vi "UI_Main.vi"(8 "error in (no error)":errorcluster, 11 "Queue Bus":T2) -> (0 "error out":errorcluster)   [LabVIEW 2020]
uses:
  Typedefs/UI_actionButton.ctl
  Typedefs/queueBus.ctl
  Typedefs/communicationData.ctl
  Typedefs/UI_controlRefs.ctl
  Typedefs/enumeratedPlayers.ctl
  Typedefs/gameState.ctl
panel:
  in  "Solve":T1
  out "Puzzle":string
  out "Cash 3":dbl caption="Player 3 cash"
  out "Cash 2":dbl caption="Player 2 cash"
  out "Cash":dbl caption="dddd cash"
  in  "buyVowel":T1
  in  "spin":T1
  out "P3_LED":bool caption="Player 3"
  out "P2_LED":bool caption="Player 2"
  in  "e-stop":bool
  out "P1_LED":bool caption="dddd"
  # "ctrl+x to quit"
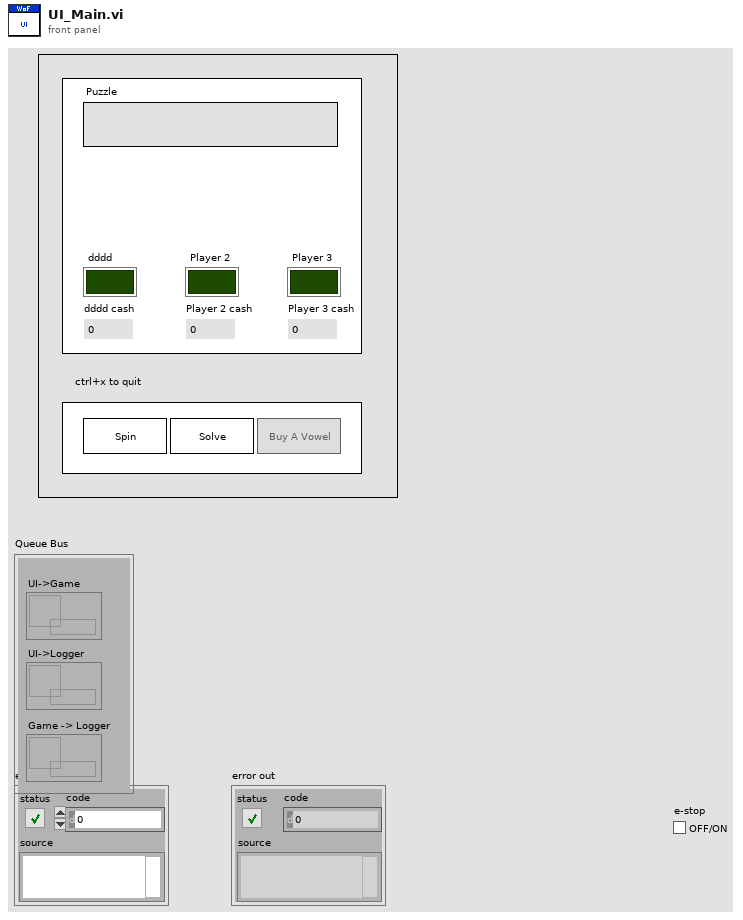
[diagram p1: front panel]
types:
  T1 = typedef "UI_actionButton.ctl" = bool
  T2 = typedef "queueBus.ctl" = cluster{"UI->Game":refnum<queue>, "UI->Logger":refnum<queue>, "Game -> Logger":refnum<queue>}
  T3 = typedef "UI_controlRefs.ctl" = cluster{"spin":refnum<vi>, "buyVowel":refnum<vi>, "Puzzle":refnum<vi>}
  T4 = typedef "communicationData.ctl" = cluster{"command":string, "payload":variant, "response":variant}
  T5 = typedef "enumeratedPlayers.ctl" = enum16{"one", "two", "three"}
  T6 = typedef "gameState.ctl" = cluster{"active player":T5, "Winnings":dbl[], "Vowel Enabled?":bool, "Puzzle State":string, "Puzzle Solved?":bool}
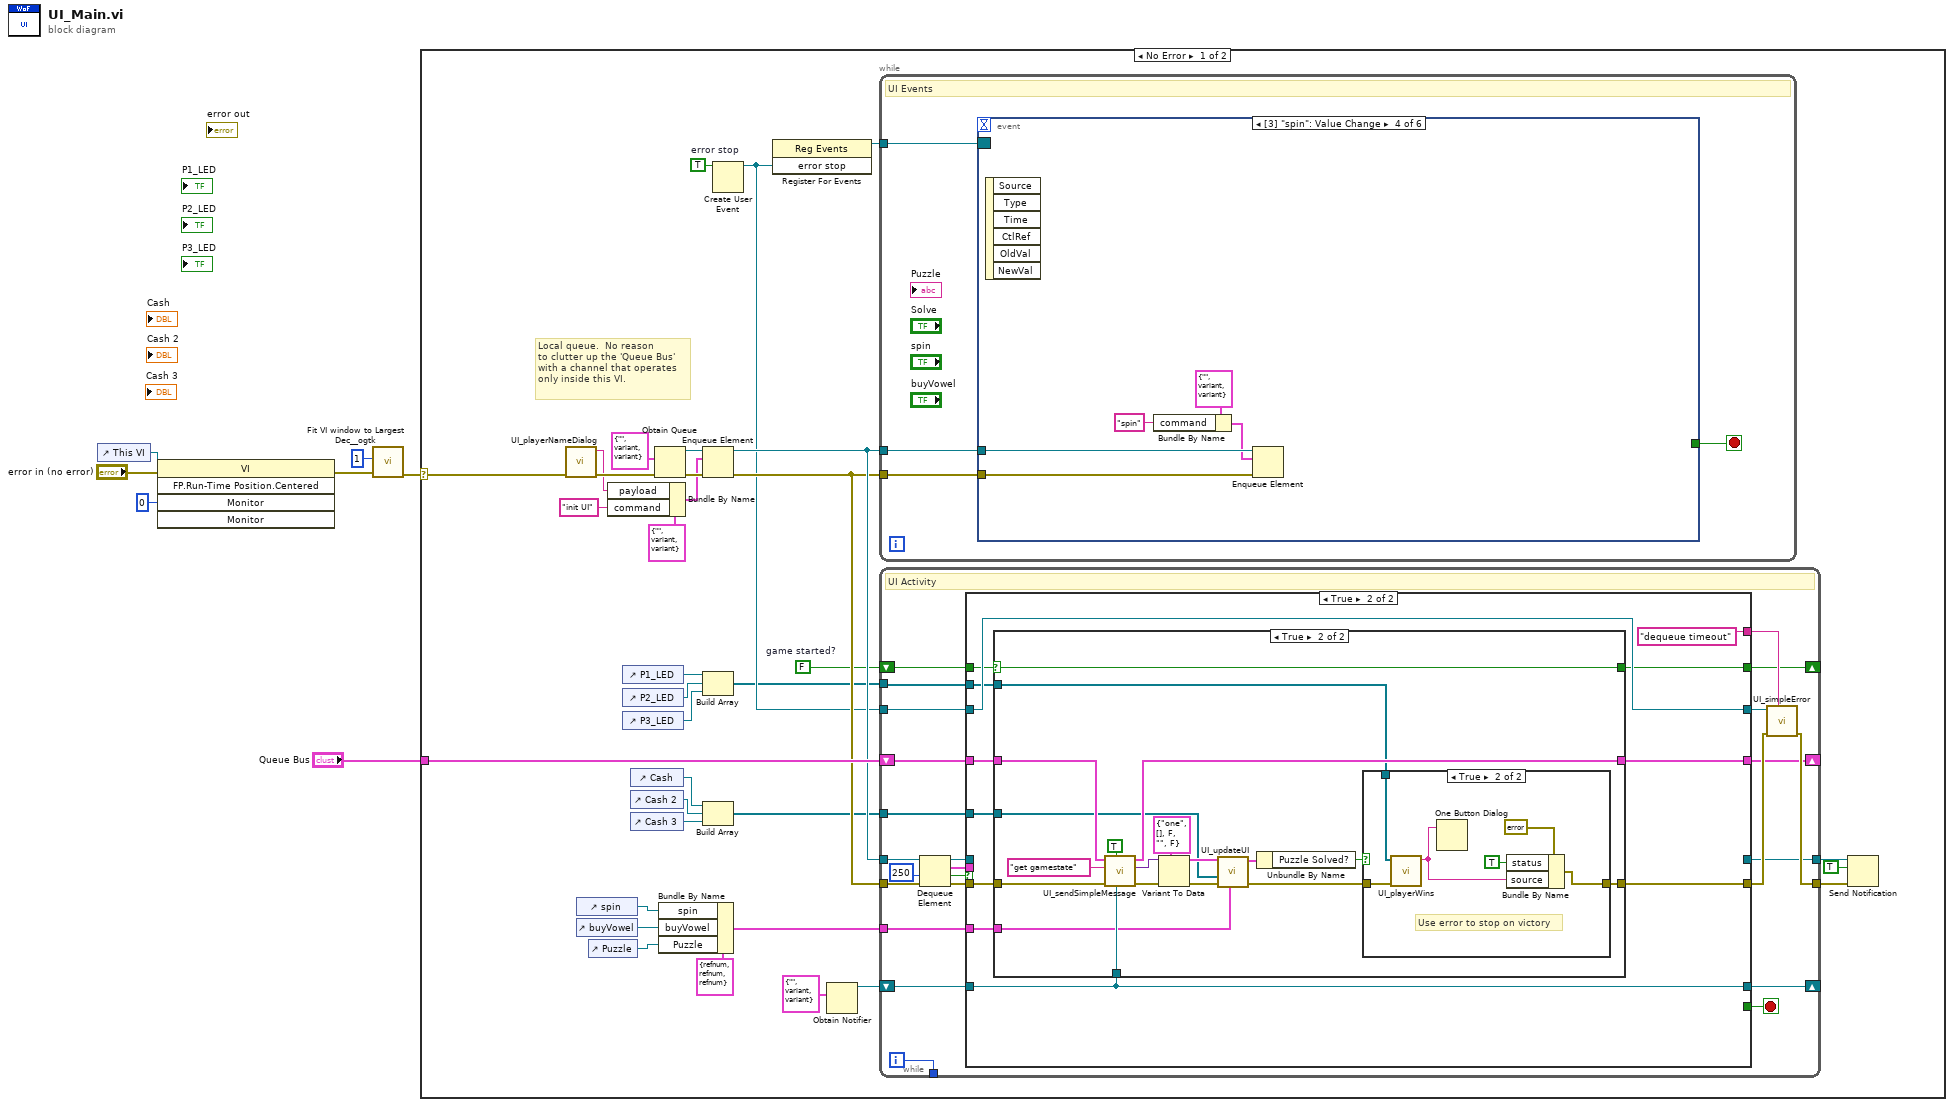
[diagram p0: block diagram]
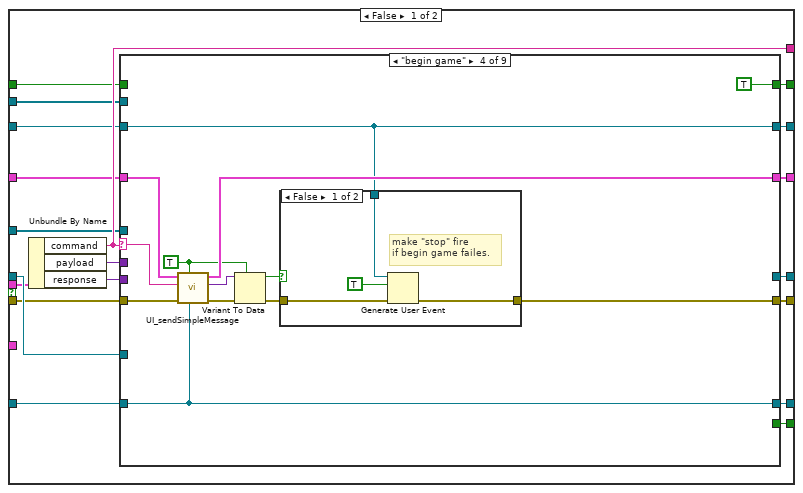
[diagram p2: hidden frame]
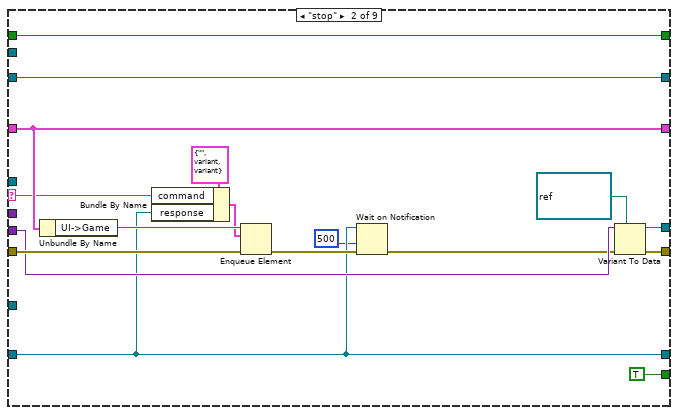
[diagram p4: hidden frame]
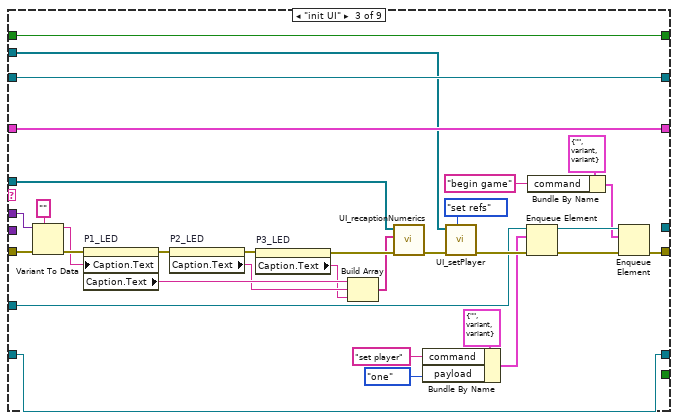
[diagram p5: hidden frame]
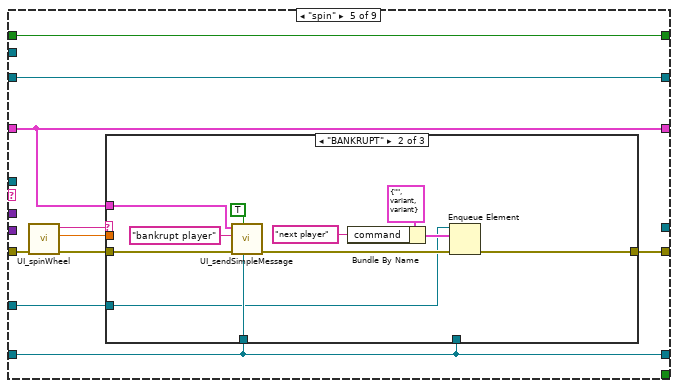
[diagram p7: hidden frame]
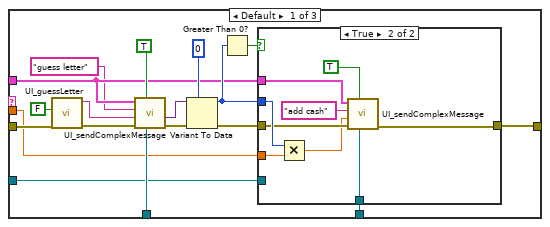
[diagram p8: hidden frame]
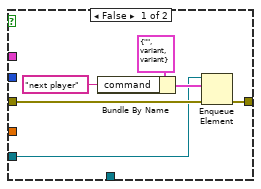
[diagram p9: hidden frame]
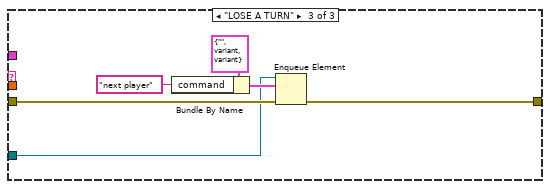
[diagram p10: hidden frame]
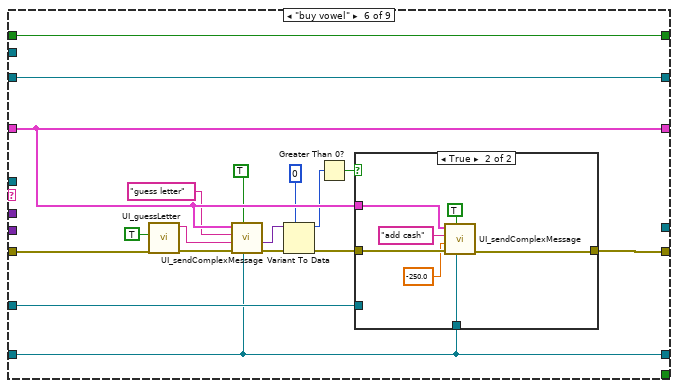
[diagram p11: hidden frame]
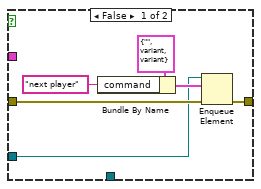
[diagram p12: hidden frame]
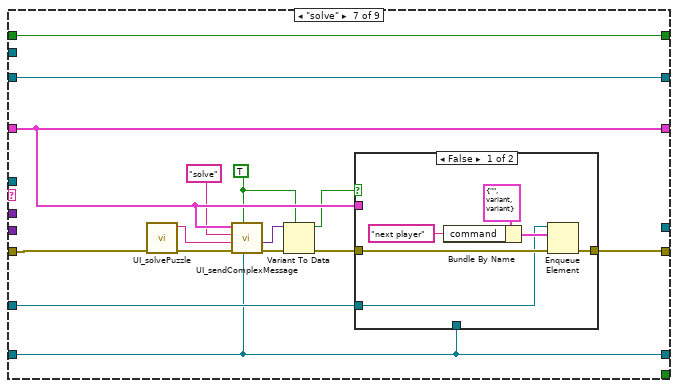
[diagram p13: hidden frame]
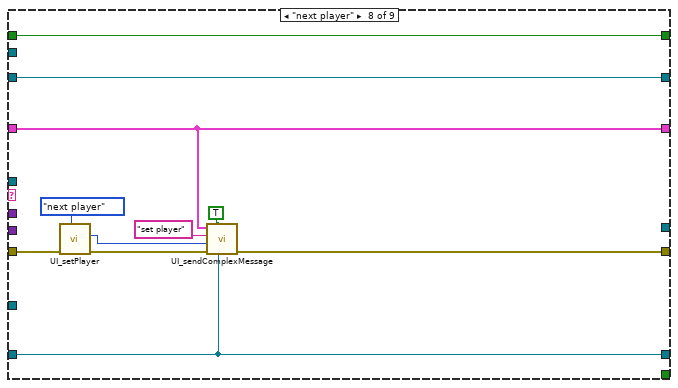
[diagram p15: hidden frame]
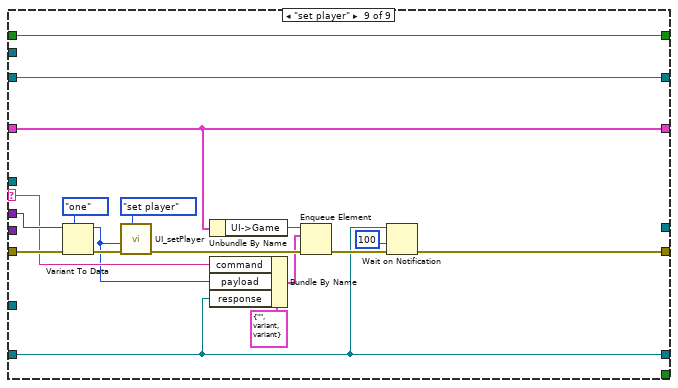
[diagram p16: hidden frame]
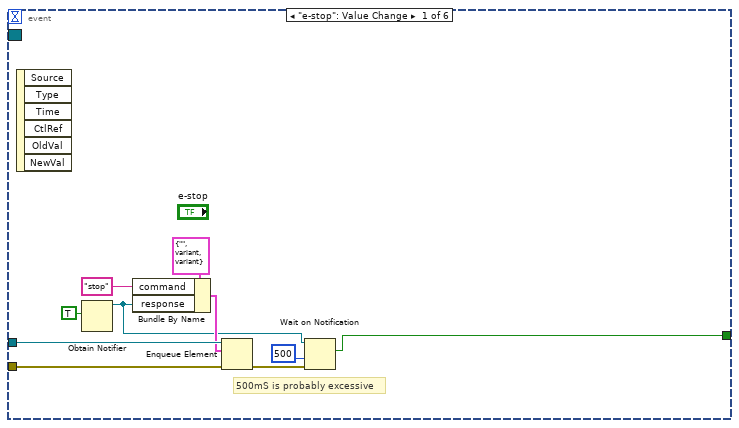
[diagram p19: hidden frame]
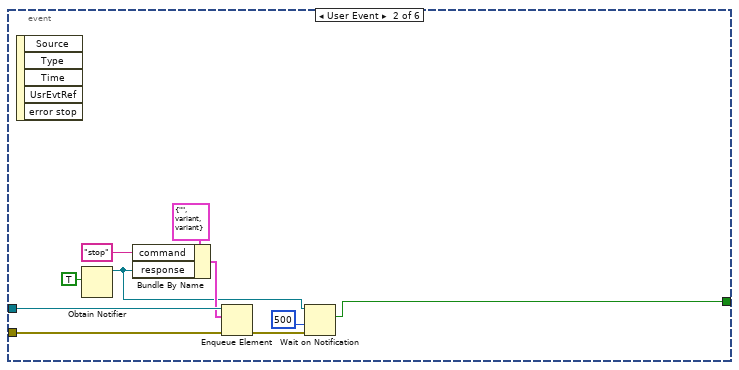
[diagram p20: hidden frame]
diagram:
  n1 = control-ref of="This VI"() -> (w2:refnum<vi>)
  n2 = invoke class="VI" method="FP.Run-Time Position.Centered"(reference=w2, error in="error in (no error)", "Monitor"=i16 0) -> (error out=w3:errorcluster)  [unwired: 2 in, 4 out]
  n3 = call <userlib>:"Fit VI window to Largest Dec__ogtk.vi"("error in (no error)"=w3, "border spacing (2 px)"=1) -> ("error out"=w5:errorcluster)  [unwired: 4 in, 1 out]
  n4 = case shown="No Error" w5 {
    selector: w5 -> [w41 _]
    tunnel: "Queue Bus" -> [w35 _]
    frame No Error {
      w17 = FALSE  # game started?
      w25 = TRUE  # error stop
      # "Local queue.  No reason\nto clutter up the 'Queue Bus'\nwith a channel that operates\nonly inside this VI."
      n5 = call "UI_playerNameDialog.vi"("error in (no error)"=w41) -> ("error out"=w40:errorcluster, "String OUT"=w29:string)  [unwired: 9 in]
      n6 = control-ref of="spin"() -> (w11:refnum<vi>)
      n7 = control-ref of="buyVowel"() -> (w10:refnum<vi>)
      n8 = control-ref of="Puzzle"() -> (w9:refnum<vi>)
      n9 = Bundle By Name(cluster=T4 {"command"="", "payload"=variant, "response"=variant} ("communication"), "payload"=w29, "command"="init UI") -> (w28:T4)
      n10 = control-ref of="P1_LED"() -> (w19:refnum<vi>)
      n11 = control-ref of="P2_LED"() -> (w20:refnum<vi>)
      n12 = control-ref of="P3_LED"() -> (w21:refnum<vi>)
      n13 = control-ref of="Cash"() -> (w16:refnum<vi>)
      n14 = control-ref of="Cash 2"() -> (w15:refnum<vi>)
      n15 = control-ref of="Cash 3"() -> (w14:refnum<vi>)
      n16 = Obtain Queue(element data type=T4 {"command"="", "payload"=variant, "response"=variant} ("communication"), error in (no error)=w40) -> (queue out=w38:refnum<queue>, error out=w33:errorcluster)  [unwired: 3 in, 1 out]
      n17 = Bundle By Name(cluster=T3 {"spin"=refnum, "buyVowel"=refnum, "Puzzle"=refnum} ("UI_controlRefs"), "spin"=w11, "buyVowel"=w10, "Puzzle"=w9) -> (w8:T3)
      n18 = Enqueue Element(queue=w38, element=w28, error in (no error)=w33) -> (queue out=w34:refnum<queue>, error out=w32:errorcluster)  [unwired: 1 in, 1 out]
      n19 = Build Array(w19, w20, w21) -> (w18:refnum<vi>[])
      n20 = Build Array(w16, w15, w14) -> (w13:refnum<vi>[])
      n21 = Create User Event(user event datatype=w25) -> (user event=w23:refnum<user-event>)  [unwired: 1 in, 1 out]
      n22 = register-events(w23) -> (reference out=w24:refnum<event-registration>)  [unwired: 2 in, 1 out]
      n23 = Obtain Notifier(notification data type=T4 {"command"="", "payload"=variant, "response"=variant} ("communication")) -> (notifier out=w26:refnum<notifier>)  [unwired: 3 in, 2 out]
      n24 = while {
        tunnel: w32 -> [w341]
        tunnel: w34 -> [w342]
        tunnel: w24 -> [w340]
        stop <- w343 stop-if-true
        # "UI Events"
        n25 = event shown="[3] \"spin\": Value Change" {
          selector: w340 -> [_ _ _ _ _ _]
          dyn-events: _ -> [_ _ _ _ _ _]
          timeout: _ -> [_ _ _ _ _ _]
          tunnel: [w344 w354 w365 _ _ _] -> w343
          tunnel: w342 -> [w353 w363 w373 w388 w393 w398]
          tunnel: w341 -> [w352 w362 w372 w387 w392 w397]
          event "e-stop": Value Change {
            # "500mS is probably excessive"
            n26 = event-data() -> ()  [unwired: 1 in, 6 out]
            n27 = Obtain Notifier(notification data type=TRUE) -> (notifier out=w346:refnum<notifier>)  [unwired: 3 in, 2 out]
            n28 = Bundle By Name(cluster=T4 {"command"="", "payload"=variant, "response"=variant} ("communication"), "command"="stop", "response"=w346) -> (w349:T4)
            n29 = Enqueue Element(queue=w353, element=w349, error in (no error)=w352) -> (error out=w347:errorcluster)  [unwired: 1 in, 2 out]
            n30 = Wait on Notification(notifier=w346, timeout in ms (-1)=500, error in (no error)=w347) -> (notification=w344:bool)  [unwired: 1 in, 3 out]
          }
          event User Event {
            n31 = event-data() -> ()  [unwired: 1 in, 5 out]
            n32 = Obtain Notifier(notification data type=TRUE) -> (notifier out=w356:refnum<notifier>)  [unwired: 3 in, 2 out]
            n33 = Bundle By Name(cluster=T4 {"command"="", "payload"=variant, "response"=variant} ("communication"), "command"="stop", "response"=w356) -> (w359:T4)
            n34 = Enqueue Element(queue=w363, element=w359, error in (no error)=w362) -> (error out=w357:errorcluster)  [unwired: 1 in, 2 out]
            n35 = Wait on Notification(notifier=w356, timeout in ms (-1)=500, error in (no error)=w357) -> (notification=w354:bool)  [unwired: 1 in, 3 out]
          }
          event Key Down? {
            n36 = event-data() -> ("Char"=w370:i16, "Mods"=w371:cluster{"Num Pad":bool, "Menu Key":bool})  [unwired: 1 in, 6 out]
            n37 = Unbundle By Name(w371) -> ("Menu Key"=w368:bool)
            n38 = Equal?(x=i16 120, y=w370) -> (x = y?=w367:bool)
            n39 = And(x=w367, y=w368) -> (x .and. y?=w364:bool)
            n40 = case shown="True" w364 {
              tunnel: w373 -> [_ w383]
              tunnel: w372 -> [_ w382]
              tunnel: [_ w381] -> w365
              frame False {
              }
              frame True {
                n41 = Obtain Notifier(notification data type=TRUE) -> (notifier out=w375:refnum<notifier>)  [unwired: 3 in, 2 out]
                n42 = Bundle By Name(cluster=T4 {"command"="", "payload"=variant, "response"=variant} ("communication"), "command"="stop", "response"=w375) -> (w378:T4)
                n43 = Enqueue Element(queue=w383, element=w378, error in (no error)=w382) -> (error out=w376:errorcluster)  [unwired: 1 in, 2 out]
                n44 = Wait on Notification(notifier=w375, timeout in ms (-1)=500, error in (no error)=w376) -> (notification=w381:bool)  [unwired: 1 in, 3 out]
              }
            }
            n45 = Not(x=w364) -> (.not. x?=w366:bool)
            n46 = event-data("Discard?"=w366) -> ()  [unwired: 1 in, 1 out]
          }
          event Value Change {
            n47 = event-data() -> ()  [unwired: 1 in, 6 out]
            n48 = Bundle By Name(cluster=T4 {"command"="", "payload"=variant, "response"=variant} ("communication"), "command"="spin") -> (w384:T4)
            n49 = Enqueue Element(queue=w388, element=w384, error in (no error)=w387) -> ()  [unwired: 1 in, 3 out]
          }
          event Value Change {
            n50 = event-data() -> ()  [unwired: 1 in, 6 out]
            n51 = Bundle By Name(cluster=T4 {"command"="", "payload"=variant, "response"=variant} ("communication"), "command"="buy vowel") -> (w389:T4)
            n52 = Enqueue Element(queue=w393, element=w389, error in (no error)=w392) -> ()  [unwired: 1 in, 3 out]
          }
          event Value Change {
            n53 = event-data() -> ()  [unwired: 1 in, 6 out]
            n54 = Bundle By Name(cluster=T4 {"command"="", "payload"=variant, "response"=variant} ("communication"), "command"="solve") -> (w394:T4)
            n55 = Enqueue Element(queue=w398, element=w394, error in (no error)=w397) -> ()  [unwired: 1 in, 3 out]
          }
        }
      }
      n56 = while {
        tunnel: w34 -> [w63]
        tunnel: w32 -> [w62]
        tunnel: [w57] -> w37
        shift-right: [w54] -> _
        shift-left: w35 -> [w55]
        shift-right: [w51] -> _
        shift-left: w26 -> [w52]
        tunnel: w23 -> [w50]
        tunnel: [w65] -> w22
        tunnel: w18 -> [w47]
        shift-right: [w46] -> _
        shift-left: w17 -> [w45]
        tunnel: [w44] -> _
        tunnel: w13 -> [w43]
        tunnel: w8 -> [w42]
        i -> [w44]
        stop <- w56 stop-if-true
        # "UI Activity"
        n57 = Dequeue Element(queue=w63, timeout in ms (-1)=250, error in (no error)=w62) -> (queue out=w53:refnum<queue>, element=w59:T4, timed out?=w60:bool, error out=w58:errorcluster)
        n58 = case shown="True" w60 {
          tunnel: w59 -> [w82 _]
          tunnel: w58 -> [w79 w305]
          tunnel: [w78 _] -> w57
          tunnel: [w77 _] -> w56
          tunnel: w55 -> [w76 w307]
          tunnel: [w75 w306] -> w54
          tunnel: w53 -> [w83 _]
          tunnel: w52 -> [w74 w301]
          tunnel: [w73 w301] -> w51
          tunnel: w50 -> [w72 w309]
          tunnel: [w71 w304] -> w64
          tunnel: [w70 w309] -> w49
          tunnel: [w84 "dequeue timeout" ("command")] -> w48
          tunnel: w47 -> [w69 w300]
          tunnel: [w68 w303] -> w46
          tunnel: w45 -> [w67 w308]
          tunnel: w43 -> [w66 w302]
          tunnel: w42 -> [_ w299]
          frame False {
            # "Item dequeued"
            n59 = Unbundle By Name(w82) -> ("command"=w84:string, "payload"=w81:variant, "response"=w80:variant)
            n60 = case shown="\"begin game\"" w84 {
              selector: w84 -> [_ w94 _ w148 _ _ _ _ w290]
              tunnel: w81 -> [_ _ w136 _ _ _ _ _ w297]
              tunnel: w80 -> [_ w99 _ _ _ _ _ _ _]
              tunnel: w79 -> [w86 w105 w137 w150 w164 w232 w252 w278 w298]
              tunnel: [_ w104 _ _ _ _ _ _ _] -> w78
              tunnel: [_ TRUE _ _ _ _ _ _ _] -> w77
              tunnel: w76 -> [w89 w98 w138 w147 w158 w229 w258 w274 w293]
              tunnel: [w89 w98 w138 w146 w158 w229 w258 w274 w293] -> w75
              tunnel: w83 -> [_ _ w122 _ w160 w231 w260 _ _]
              tunnel: w74 -> [w88 w91 w112 w145 w157 w228 w257 w273 w285]
              tunnel: [w88 w91 w112 w145 w157 w228 w257 w273 w285] -> w73
              tunnel: w72 -> [w87 w102 w111 w140 w166 w234 w262 w280 w282]
              tunnel: [w86 w101 w110 w139 w159 w230 w259 w270 w283] -> w71
              tunnel: [w87 w102 w111 w140 w166 w234 w262 w280 w282] -> w70
              tunnel: w69 -> [_ _ w109 _ _ _ _ _ _]
              tunnel: [w85 w100 w108 TRUE w165 w233 w261 w279 w281] -> w68
              tunnel: w67 -> [w85 w100 w108 _ w165 w233 w261 w279 w281]
              tunnel: w66 -> [_ _ w107 _ _ _ _ _ _]
              frame Default {
              }
              frame "stop" {
                n61 = Unbundle By Name(w98) -> ("UI->Game"=w96:refnum<queue>)
                n62 = Bundle By Name(cluster=T4 {"command"="", "payload"=variant, "response"=variant} ("communication"), "command"=w94, "response"=w91) -> (w93:T4)
                n63 = Enqueue Element(queue=w96, element=w93, error in (no error)=w105) -> (error out=w97:errorcluster)  [unwired: 1 in, 2 out]
                n64 = Wait on Notification(notifier=w91, timeout in ms (-1)=500, error in (no error)=w97) -> (error out=w92:errorcluster)  [unwired: 1 in, 3 out]
                n65 = Variant To Data(error in=w92, type=refnum<notifier> refnum ("notifier out"), Variant=w99) -> (data=w104:refnum<notifier>, error out=w101:errorcluster)
              }
              frame "init UI" {
                n66 = Variant To Data(error in=w137, type="", Variant=w136) -> (data=w133:string, error out=w134:errorcluster)
                n67 = property on="P1_LED" class="Bool (strict)"(error in=w134, "Caption.Text"=w133) -> (error out=w132:errorcluster, "Caption.Text"=w130:string)  [unwired: 1 in, 1 out]
                n68 = property on="P2_LED" class="Bool (strict)"(error in=w132) -> (error out=w131:errorcluster, "Caption.Text"=w129:string)  [unwired: 1 in, 1 out]
                n69 = property on="P3_LED" class="Bool (strict)"(error in=w131) -> (error out=w127:errorcluster, "Caption.Text"=w128:string)  [unwired: 1 in, 1 out]
                n70 = Build Array(w130, w129, w128) -> (w126:string[])
                n71 = call "UI_recaptionNumerics.vi"("error in (no error)"=w127, "Names"=w126, "Numeric Refs"=w107) -> ("error out"=w125:errorcluster)  [unwired: 8 in]
                n72 = Bundle By Name(cluster=T4 {"command"="", "payload"=variant, "response"=variant} ("communication"), "command"="set player", "payload"=enum16{"one", "two", "three"}."one" ("player")) -> (w119:T4)
                n73 = call "UI_setPlayer.vi"("action"=enum16{"set refs", "set player", "next player"}."set refs", "error in (no error)"=w125, "LED refs"=w109) -> ("error out"=w123:errorcluster)  [unwired: 7 in, 1 out]
                n74 = Enqueue Element(queue=w122, element=w119, error in (no error)=w123) -> (queue out=w118:refnum<queue>, error out=w117:errorcluster)  [unwired: 1 in, 1 out]
                n75 = Bundle By Name(cluster=T4 {"command"="", "payload"=variant, "response"=variant} ("communication"), "command"="begin game") -> (w113:T4)
                n76 = Enqueue Element(queue=w118, element=w113, error in (no error)=w117) -> (error out=w110:errorcluster)  [unwired: 1 in, 2 out]
              }
              frame "begin game" {
                w143 = TRUE ("Wait for Response")
                n77 = call "UI_sendSimpleMessage.vi"("notifier"=w145, "Wait for Response"=w143, "error in (no error)"=w150, "Command"=w148, "Queue Bus"=w147) -> ("error out"=w149:errorcluster, "payload"=w144:variant, "Queue Bus OUT"=w146:T2)  [unwired: 4 in]
                n78 = Variant To Data(error in=w149, type=w143, Variant=w144) -> (data=w141:bool, error out=w142:errorcluster)
                n79 = case shown="False" w141 {
                  tunnel: w142 -> [w155 w156]
                  tunnel: w140 -> [w154 _]
                  tunnel: [w152 w156] -> w139
                  frame False {
                    # "make \"stop\" fire\nif begin game failes."
                    n80 = Generate User Event(user event=w154, event data cluster=TRUE ("event data"), error in=w155) -> (error out=w152:errorcluster)  [unwired: 1 in, 1 out]
                  }
                  frame True {
                  }
                }
              }
              frame "spin" {
                n81 = call "UI_spinWheel.vi"("error in (no error)"=w164) -> ("error out"=w161:errorcluster, "Cash"=w162:dbl, "Spin Result"=w163:string)  [unwired: 8 in]
                n82 = case shown="\"BANKRUPT\"" w163 {
                  tunnel: w162 -> [w171 _ _]
                  tunnel: w161 -> [w184 w210 w216]
                  tunnel: w160 -> [w174 w201 w212]
                  tunnel: [w173 w200 w211] -> w159
                  tunnel: w158 -> [w170 w209 _]
                  tunnel: w157 -> [w181 w207 _]
                  tunnel: w157 -> [w168 _ _]
                  frame Default {
                    n83 = call "UI_guessLetter.vi"("error in (no error)"=w184, "buyingVowel?"=FALSE) -> ("error out"=w183:errorcluster, "Letter OUT"=w180:string)  [unwired: 8 in]
                    n84 = call "UI_sendComplexMessage.vi"("notifier"=w181, "Wait for Response"=TRUE, "error in (no error)"=w183, "Payload"=w180, "Command"="guess letter", "Queue Bus"=w170) -> ("error out"=w182:errorcluster, "payload"=w178:variant)  [unwired: 3 in, 1 out]
                    n85 = Variant To Data(error in=w182, type=0, Variant=w178) -> (data=w172:i32, error out=w175:errorcluster)
                    n86 = Greater Than 0?(x=w172) -> (x > 0?=w176:bool)
                    n87 = case shown="True" w176 {
                      tunnel: w175 -> [w187 w197]
                      tunnel: w174 -> [w185 _]
                      tunnel: [w186 w191] -> w173
                      tunnel: w172 -> [_ w198]
                      tunnel: w171 -> [_ w199]
                      tunnel: w170 -> [_ w195]
                      tunnel: w168 -> [_ w196]
                      frame False {
                        n88 = Bundle By Name(cluster=T4 {"command"="", "payload"=variant, "response"=variant} ("communication"), "command"="next player") -> (w188:T4)
                        n89 = Enqueue Element(queue=w185, element=w188, error in (no error)=w187) -> (error out=w186:errorcluster)  [unwired: 1 in, 2 out]
                      }
                      frame True {
                        n90 = Multiply(x=w198, y=w199) -> (x*y=w193:dbl)
                        n91 = call "UI_sendComplexMessage.vi"("notifier"=w196, "Wait for Response"=TRUE, "error in (no error)"=w197, "Payload"=w193, "Command"="add cash", "Queue Bus"=w195) -> ("error out"=w191:errorcluster)  [unwired: 3 in, 2 out]
                      }
                    }
                  }
                  frame "BANKRUPT" {
                    n92 = call "UI_sendSimpleMessage.vi"("notifier"=w207, "Wait for Response"=TRUE, "error in (no error)"=w210, "Command"="bankrupt player", "Queue Bus"=w209) -> ("error out"=w202:errorcluster)  [unwired: 4 in, 2 out]
                    n93 = Bundle By Name(cluster=T4 {"command"="", "payload"=variant, "response"=variant} ("communication"), "command"="next player") -> (w203:T4)
                    n94 = Enqueue Element(queue=w201, element=w203, error in (no error)=w202) -> (error out=w200:errorcluster)  [unwired: 1 in, 2 out]
                  }
                  frame "LOSE A TURN" {
                    n95 = Bundle By Name(cluster=T4 {"command"="", "payload"=variant, "response"=variant} ("communication"), "command"="next player") -> (w213:T4)
                    n96 = Enqueue Element(queue=w212, element=w213, error in (no error)=w216) -> (error out=w211:errorcluster)  [unwired: 1 in, 2 out]
                  }
                }
              }
              frame "buy vowel" {
                n97 = call "UI_guessLetter.vi"("error in (no error)"=w232, "buyingVowel?"=TRUE) -> ("error out"=w227:errorcluster, "Letter OUT"=w225:string)  [unwired: 8 in]
                n98 = call "UI_sendComplexMessage.vi"("notifier"=w228, "Wait for Response"=TRUE, "error in (no error)"=w227, "Payload"=w225, "Command"="guess letter", "Queue Bus"=w229) -> ("error out"=w226:errorcluster, "payload"=w223:variant)  [unwired: 3 in, 1 out]
                n99 = Variant To Data(error in=w226, type=0, Variant=w223) -> (data=w219:i32, error out=w220:errorcluster)
                n100 = Greater Than 0?(x=w219) -> (x > 0?=w221:bool)
                n101 = case shown="True" w221 {
                  tunnel: w220 -> [w237 w247]
                  tunnel: w231 -> [w235 _]
                  tunnel: [w236 w242] -> w230
                  tunnel: w229 -> [_ w245]
                  tunnel: w228 -> [_ w246]
                  frame False {
                    n102 = Bundle By Name(cluster=T4 {"command"="", "payload"=variant, "response"=variant} ("communication"), "command"="next player") -> (w238:T4)
                    n103 = Enqueue Element(queue=w235, element=w238, error in (no error)=w237) -> (error out=w236:errorcluster)  [unwired: 1 in, 2 out]
                  }
                  frame True {
                    n104 = call "UI_sendComplexMessage.vi"("notifier"=w246, "Wait for Response"=TRUE, "error in (no error)"=w247, "Payload"=-250.0 ("Cash"), "Command"="add cash", "Queue Bus"=w245) -> ("error out"=w242:errorcluster)  [unwired: 3 in, 2 out]
                  }
                }
              }
              frame "solve" {
                w249 = TRUE ("Wait for Response")
                n105 = call "UI_solvePuzzle.vi"("error in (no error)"=w252) -> ("error out"=w251:errorcluster, "String OUT"=w250:string)  [unwired: 9 in]
                n106 = call "UI_sendComplexMessage.vi"("notifier"=w257, "Wait for Response"=w249, "error in (no error)"=w251, "Payload"=w250, "Command"="solve", "Queue Bus"=w258) -> ("error out"=w256:errorcluster, "payload"=w255:variant)  [unwired: 3 in, 1 out]
                n107 = Variant To Data(error in=w256, type=w249, Variant=w255) -> (data=w248:bool, error out=w254:errorcluster)
                n108 = case shown="False" w248 {
                  tunnel: w254 -> [w265 w269]
                  tunnel: w260 -> [w263 _]
                  tunnel: [w264 w269] -> w259
                  tunnel: w258 -> [_ _]
                  tunnel: w257 -> [_ _]
                  frame False {
                    n109 = Bundle By Name(cluster=T4 {"command"="", "payload"=variant, "response"=variant} ("communication"), "command"="next player") -> (w266:T4)
                    n110 = Enqueue Element(queue=w263, element=w266, error in (no error)=w265) -> (error out=w264:errorcluster)  [unwired: 1 in, 2 out]
                  }
                  frame True {
                  }
                }
              }
              frame "next player" {
                n111 = call "UI_setPlayer.vi"("action"=enum16{"set refs", "set player", "next player"}."next player", "error in (no error)"=w278) -> ("error out"=w276:errorcluster, "Player"=w275:i32)  [unwired: 8 in]
                n112 = call "UI_sendComplexMessage.vi"("notifier"=w273, "Wait for Response"=TRUE, "error in (no error)"=w276, "Payload"=w275, "Command"="set player", "Queue Bus"=w274) -> ("error out"=w270:errorcluster)  [unwired: 3 in, 2 out]
              }
              frame "set player" {
                n113 = Variant To Data(error in=w298, type=enumeratedPlayers."one" ("player"), Variant=w297) -> (data=w289:T5, error out=w295:errorcluster)
                n114 = call "UI_setPlayer.vi"("action"=enum16{"set refs", "set player", "next player"}."set player", "error in (no error)"=w295, "player"=w289) -> ("error out"=w288:errorcluster)  [unwired: 7 in, 1 out]
                n115 = Unbundle By Name(w293) -> ("UI->Game"=w292:refnum<queue>)
                n116 = Bundle By Name(cluster=T4 {"command"="", "payload"=variant, "response"=variant} ("communication"), "command"=w290, "payload"=w289, "response"=w285) -> (w287:T4)
                n117 = Enqueue Element(queue=w292, element=w287, error in (no error)=w288) -> (error out=w286:errorcluster)  [unwired: 1 in, 2 out]
                n118 = Wait on Notification(notifier=w285, timeout in ms (-1)=100, error in (no error)=w286) -> (error out=w283:errorcluster)  [unwired: 1 in, 3 out]
              }
            }
          }
          frame True {
            # "Dequeue timed out"
            n119 = case shown="True" w308 {
              selector: w308 -> [w311 w332]
              tunnel: w307 -> [w313 w330]
              tunnel: [w313 w329] -> w306
              tunnel: w305 -> [w312 w331]
              tunnel: [w312 w314] -> w304
              tunnel: [w311 w332] -> w303
              tunnel: w302 -> [_ w319]
              tunnel: w301 -> [_ w328]
              tunnel: w300 -> [_ w315]
              tunnel: w299 -> [_ w321]
              frame False {
              }
              frame True {
                n120 = call "UI_sendSimpleMessage.vi"("notifier"=w328, "Wait for Response"=TRUE, "error in (no error)"=w331, "Command"="get gamestate", "Queue Bus"=w330) -> ("error out"=w325:errorcluster, "payload"=w324:variant, "Queue Bus OUT"=w329:T2)  [unwired: 4 in]
                n121 = Variant To Data(error in=w325, type=T6 {"active player"=enum."one", "Winnings"=[], "Vowel Enabled?"=FALSE, "Puzzle State"="", "Puzzle Solved?"=FALSE} ("gameState"), Variant=w324) -> (data=w320:T6, error out=w322:errorcluster)
                n122 = call "UI_updateUI.vi"("UI_controlRefs"=w321, "error in (no error)"=w322, "Player Winnings"=w319, "Game State"=w320) -> ("error out"=w317:errorcluster, "Game State OUT"=w318:T6)  [unwired: 6 in]
                n123 = Unbundle By Name(w318) -> ("Puzzle Solved?"=w316:bool)
                n124 = case shown="True" w316 {
                  tunnel: w317 -> [w333 w339]
                  tunnel: w315 -> [_ w338]
                  tunnel: [w333 w334] -> w314
                  frame False {
                  }
                  frame True {
                    # "Use error to stop on victory"
                    n125 = call "UI_playerWins.vi"("error in (no error)"=w339, "Array"=w338) -> ("win string"=w335:string)  [unwired: 8 in, 1 out]
                    n126 = One Button Dialog(message=w335) -> ()  [unwired: 1 in, 1 out]
                    n127 = Bundle By Name(cluster=errorcluster {"status"=FALSE, "code"=0, "source"=""} ("error constant"), "status"=TRUE, "source"=w335) -> (w334:errorcluster)
                  }
                }
              }
            }
          }
        }
        n128 = call "UI_simpleError.vi"("command"=w48, "error in (no error)"=w64, "error stop"=w49) -> ("error out"=w65:errorcluster)  [unwired: 8 in]
      }
      n129 = Send Notification(notification=TRUE, notifier=w37, error in (no error)=w22) -> ()  [unwired: 2 out]
    }
    frame Error {
    }
  }
